vi "Check Password.vi"(11 "Message":string) -> (2 "Payload":string, 3 "uService ID":string)   [LabVIEW 2026, in "TALOS.lvlib" / "TCP Server.lvlib" / "TCP Server.lvclass"]
uses:
  TCP Server.lvclass
  Ancestor/Ancestor/Ancestor.lvclass/Ancestor.ctl
  Support VIs/Circus Config Param - Core.vi
  Support VIs/Generate Error.vi
  Support VIs/Circus Root Path.vi
  Support VIs/TALOS Config Param.vi
  FGV/Error Memory/Get Error Description.vi
  Support VIs/Get PC name.vi
  Ancestor/Ancestor/Read ID.vi
  Support VIs/Get Class Name.vi
  FGV/Error Memory/Error Memory Core.vi
  <vilib>/AdvancedString/Delimited String to 1D String Array.vi
  <vilib>/AdvancedString/Delimited String to 1D String Array (string).vi
  FGV/Error Memory/Error Crt Lvl checker.vi
  FGV/Error Memory/Error Memory Core.vi/40c8088d-b597-4017-91af-faa98e00292e.vi
  FGV/Error Memory/Error Memory Core.vi/d4a3ab98-063c-4e44-b43d-fbdcfe6c2be2.vi
  Support VIs/Global Memory.vi
  <vilib>/Utility/LVClass/Get LV Class Name.vi
  Support VIs/TALOS Root path.vi
  Support VIs/Read CSV worksheet.vi
  Support VIs/Global Constants.vi
  <vilib>/Utility/error.llb/General Error Handler.vi
  <vilib>/Utility/config.llb/Open Config Data.vi
  <vilib>/Utility/config.llb/Get Section Names.vi
  <vilib>/Utility/config.llb/Get Key Names.vi
  <vilib>/Utility/config.llb/Read Key.vi
  <vilib>/Utility/config.llb/Read Key (String).vi
  <vilib>/Utility/config.llb/Close Config Data.vi
  <vilib>/Utility/error.llb/Search and Replace Pattern.vi
  <vilib>/Utility/error.llb/Search and Replace Pattern (string).vi
  Ancestor/Ancestor/Ancestor.lvclass
  <vilib>/Comparison/Equal/Equal Functor/Equal Functor.lvclass
  TALOS.lvlib
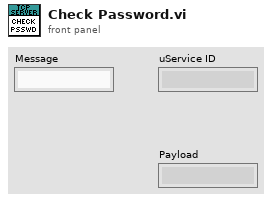
[diagram p1: front panel]
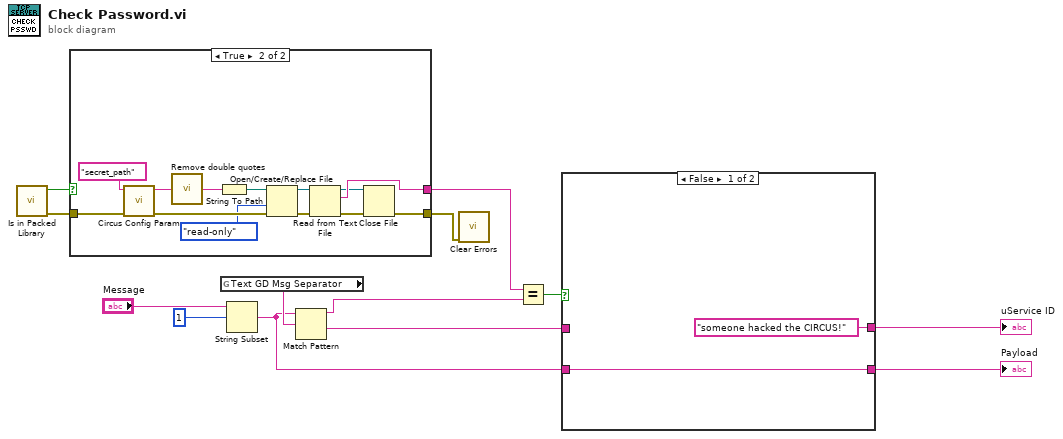
[diagram p0: block diagram]
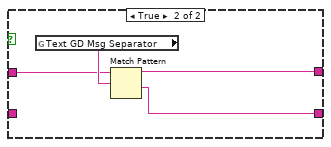
[diagram p2: hidden frame]
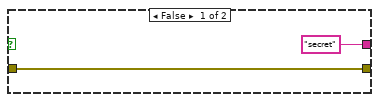
[diagram p3: hidden frame]
diagram:
  n1 = call "Is in Packed Library.vi"() -> ("error out"=w10:errorcluster, "Is In Packed Library"=w9:bool)  [unwired: 10 in]
  n2 = case shown="True" w9 {
    tunnel: w10 -> [w14 w28]
    tunnel: ["secret" ("Value") w17] -> w8
    tunnel: [w14 w25] -> w1
    frame False {
    }
    frame True {
      n3 = call "Circus Config Param.vi"("error in (no error)"=w28, "Parameter Name"="secret_path") -> ("error out"=w24:errorcluster, "Value"=w26:string)  [unwired: 8 in]
      n4 = call "Remove double quotes.vi"("Input string"=w26) -> ("Output string"=w23:string)  [unwired: 4 in]
      n5 = String To Path(string=w23) -> (path=w22:path)
      n6 = Open/Create/Replace File(file path (use dialog)=w22, error in=w24, access (0:read/write)=enum16{"read/write", "read-only", "write-only"}."read-only") -> (refnum out=w20:refnum<file>, error out=w19:errorcluster)  [unwired: 3 in, 1 out]
      n7 = Read from Text File(file (use dialog)=w20, error in=w19) -> (refnum out=w16:refnum<file>, text=w17:string, error out=w18:errorcluster)  [unwired: 2 in, 1 out]
      n8 = Close File(refnum=w16, error in=w18) -> (error out=w25:errorcluster)  [unwired: 1 out]
    }
  }
  n9 = global read "Global Constants.vi" "Text GD Msg Separator"() -> (w11:string)
  n10 = String Subset(string="Message", offset (0)=1) -> (substring=w2:string)  [unwired: 1 in]
  n11 = Match Pattern(string=w2, regular expression=w11) -> (before substring=w7:string, after substring=w5:string)  [unwired: 1 in, 2 out]
  n12 = call <vilib>:"Clear Errors.vi"("error in (no error)"=w1) -> ()  [unwired: 5 in, 2 out]
  n13 = Equal?(x=w8, y=w7) -> (x = y?=w6:bool)
  n14 = case shown="False" w6 {
    tunnel: w5 -> [_ w33]
    tunnel: ["someone hacked the CIRCUS!" ("Message") w32] -> w4
    tunnel: [w29 w31] -> w3
    tunnel: w2 -> [w29 _]
    frame False {
    }
    frame True {
      n15 = global read "Global Constants.vi" "Text GD Msg Separator"() -> (w34:string)
      n16 = Match Pattern(string=w33, regular expression=w34) -> (before substring=w32:string, after substring=w31:string)  [unwired: 1 in, 2 out]
    }
  }
  "Payload" <- w3
  "uService ID" <- w4
